vi "4CHDAQ - Enter File Name.vi"() -> (3 "String 2":string)   [LabVIEW 2015]
panel:
  in  "OK Button":bool
  in  "String":string
  # "Enter File Name"
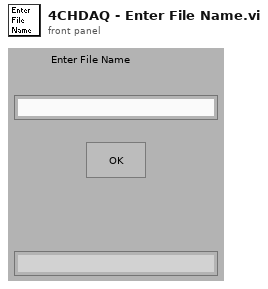
[diagram p1: front panel]
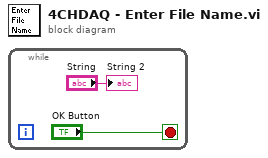
[diagram p0: block diagram]
diagram:
  n1 = while {
    stop <- "OK Button" stop-if-true
    "String 2" <- "String"
  }
